vi "SubVIs3.vi"(8 "error in (no error)":errorcluster, 10 "B":dbl[](array[numeric]), 11 "A":dbl[](array[numeric])) -> (0 "error out":errorcluster, 2 "A / B":dbl[](array[numeric]), 3 "(A x B)":dbl[](array[numeric]))   [LabVIEW 2014]
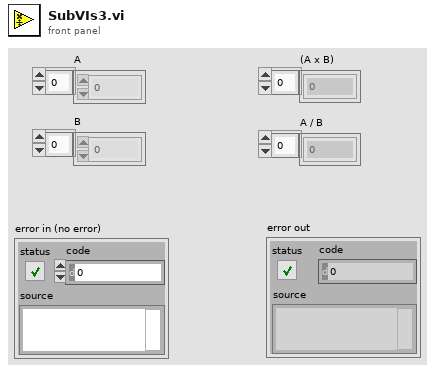
[diagram p1: front panel]
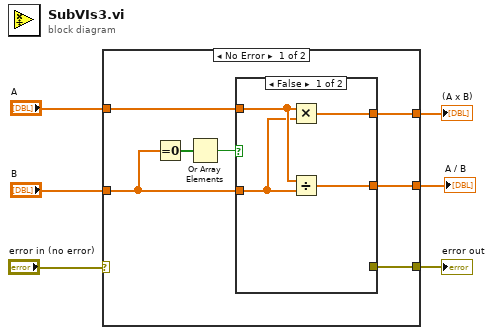
[diagram p0: block diagram]
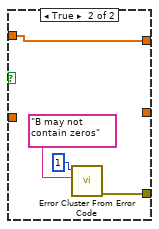
[diagram p2: hidden frame]
diagram:
  n1 = case shown="No Error" "error in (no error)" {
    selector: "error in (no error)" -> [_ w22]
    tunnel: "A" -> [w13 _]
    tunnel: [w12 _] -> w5
    tunnel: [w11 _] -> w4
    tunnel: "B" -> [w10 _]
    tunnel: [w7 w22] -> w2
    frame No Error {
      n2 = Equal To 0?(x=w10) -> (x = 0?=w9:bool[])
      n3 = Or Array Elements(Boolean array=w9) -> (logical OR=w8:bool)
      n4 = case shown="False" w8 {
        tunnel: w13 -> [w17 w21]
        tunnel: [w16 w21] -> w12
        tunnel: [w15 _] -> w11
        tunnel: w10 -> [w14 _]
        tunnel: [_ w18] -> w7
        frame False {
          n5 = Multiply(x=w17, y=w14) -> (x*y=w16:dbl[])
          n6 = Divide(x=w17, y=w14) -> (x/y=w15:dbl[])
        }
        frame True {
          n7 = call <vilib>:"Error Cluster From Error Code.vi"("error message (\"\")"="B may not contain zeros" ("error message (\"\")"), "error code (0)"=1) -> ("error out"=w18:errorcluster)  [unwired: 7 in]
        }
      }
    }
    frame Error {
    }
  }
  "(A x B)" <- w5
  "A / B" <- w4
  "error out" <- w2
